vi "readArrayFromFile.vi"(2 "error in (no error)":errorcluster, 3 "file":path) -> (0 "error out":errorcluster, 1 "array":dbl[][](array[numeric]) format="%_5f")   [LabVIEW 2014, in "Array.lvlib"]
uses:
  Array.lvlib
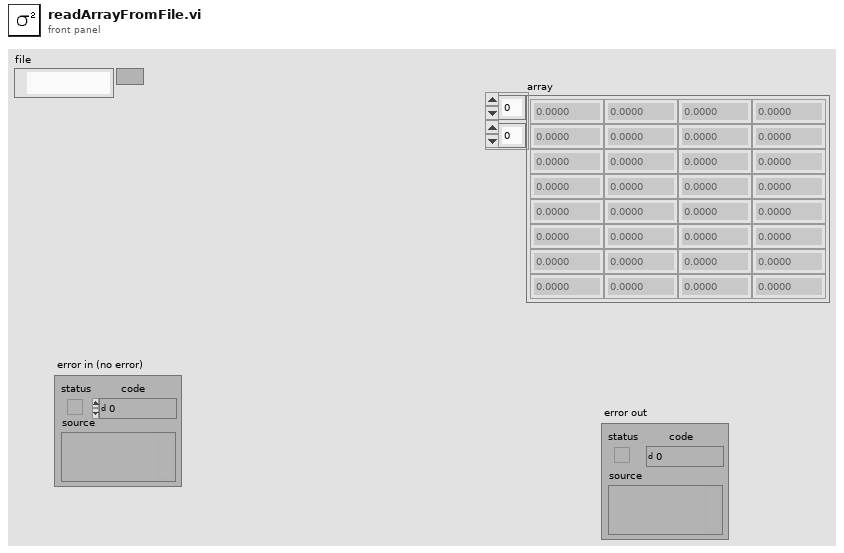
[diagram p1: front panel]
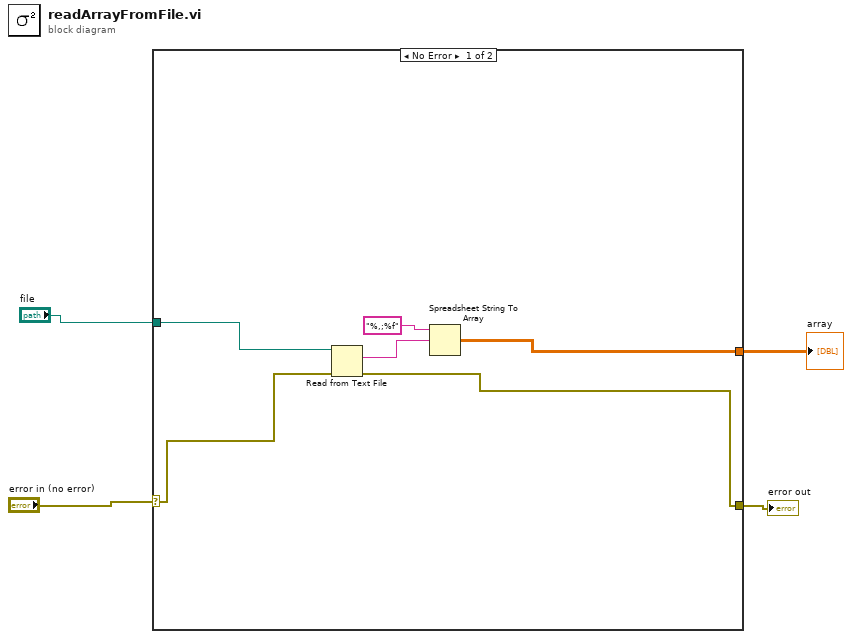
[diagram p0: block diagram]
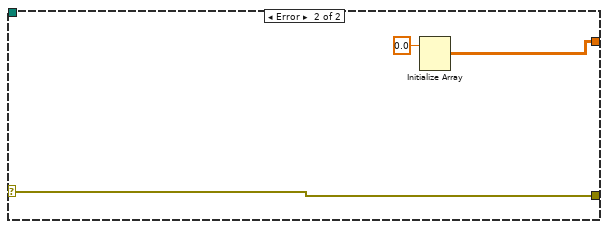
[diagram p2: hidden frame]
diagram:
  n1 = case shown="No Error" "error in (no error)" {
    selector: "error in (no error)" -> [w8 w13]
    tunnel: [w7 w13] -> w3
    tunnel: "file" -> [w9 _]
    tunnel: [w6 w12] -> w1
    frame No Error {
      n2 = Read from Text File(file (use dialog)=w9, error in=w8) -> (text=w5:string, error out=w7:errorcluster)  [unwired: 2 in, 2 out]
      n3 = Spreadsheet String To Array(format string="%,;%f", spreadsheet string=w5) -> (array=w6:dbl[][])  [unwired: 2 in]
    }
    frame Error {
      n4 = Initialize Array(0.0 ("element")) -> (w12:dbl[][])  [unwired: 2 in]
    }
  }
  "error out" <- w3
  "array" <- w1
